vi "Voltage Based Speed Control (FPGA).vi"(0 "SpeedRead":fxp<+/-,20,5>, 5 "SpeedCtrl":fxp<+/-,20,5>, 7 "Speed?":bool, 9 "VoltCtrl":fxp<+/-,20,5>, 11 "SpeedCtrlRate":i16, 12 "SpeedStep":fxp<+/-,20,5>) -> (8 "VoltCtrlOut":fxp<+/-,21,6>)   [LabVIEW 2013]
uses:
  <vilib>/rvi/FXPMathLib/FxpDiv/subVIs/nifxpmath_Div_SimConfig.ctl
  <vilib>/rvi/Emulation/niFpgaSctlEmulationGetInTimedLoop.vi
  <vilib>/rvi/Emulation/niFpgaEmulationReportErrorSimple.vi
  <vilib>/rvi/Emulation/niFpgaGetClockAttributes.vi
  <vilib>/rvi/FXPMathLib/FxpDiv/simVIs/DllFxpDivTemp_sub.vi
  <vilib>/rvi/Emulation/niFpgaCriticalErrorInLSC.vi
  <vilib>/rvi/FXPMathLib/FxpSub/XNode/nifxpmath_Sub.xnode
  <vilib>/rvi/FXPMathLib/FxpDiv/XNode/nifxpmath_Div.xnode
  <vilib>/rvi/FXPMathLib/FxpMul/XNode/nifxpmath_Multiplier.xnode
  <vilib>/rvi/FXPMathLib/FxpAdd/XNode/nifxpmath_Add.xnode
  <vilib>/rvi/FXPMathLib/sim/FxpSim.dll
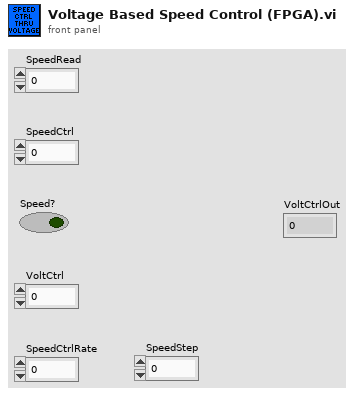
[diagram p1: front panel]
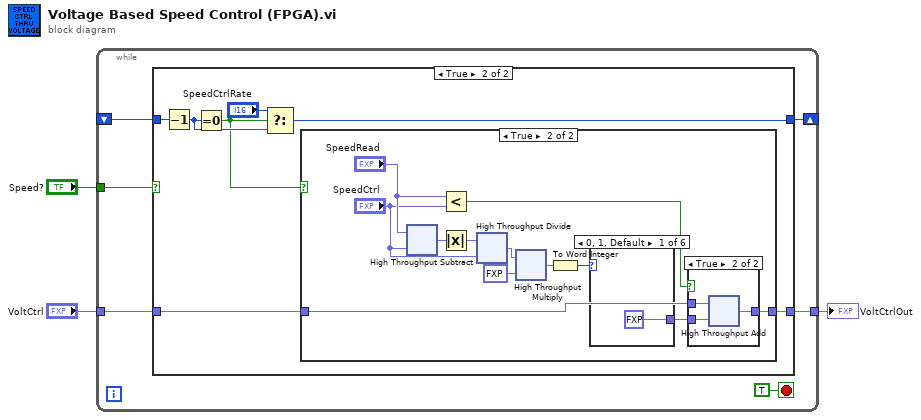
[diagram p0: block diagram]
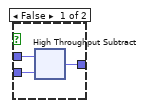
[diagram p4: hidden frame]
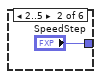
[diagram p5: hidden frame]
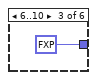
[diagram p6: hidden frame]
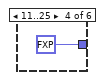
[diagram p7: hidden frame]
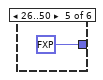
[diagram p8: hidden frame]
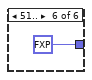
[diagram p9: hidden frame]
diagram:
  n1 = while {
    tunnel: "Speed?" -> [w9]
    tunnel: "VoltCtrl" -> [w8]
    tunnel: [w7] -> w1
    shift-right: [w4] -> _
    shift-left: _ -> [w5]
    stop <- TRUE stop-if-true
    n2 = case shown="True" w9 {
      tunnel: [w11 w12] -> w7
      tunnel: w8 -> [w11 w14]
      tunnel: w5 -> [_ w18]
      tunnel: [i16 0 ("SpeedCtrlRate") w15] -> w4
      frame False {
      }
      frame True {
        n3 = Decrement(x=w18) -> (x-1=w16:i16)
        n4 = Equal To 0?(x=w16) -> (x = 0?=w13:bool)
        n5 = Select(t="SpeedCtrlRate", s=w13, f=w16) -> (s? t:f=w15:i16)
        n6 = case shown="True" w13 {
          tunnel: w14 -> [w19 w21]
          tunnel: [w19 w22] -> w12
          frame False {
          }
          frame True {
            n7 = xnode "High Throughput Subtract"("x"="SpeedRead", "y"="SpeedCtrl") -> ("x-y"=w30:fxp<+/-,21,6>)
            n8 = Less?(x="SpeedRead", y="SpeedCtrl") -> (x < y?=w23:bool)
            n9 = Absolute Value(x=w30) -> (abs(x)=w29:fxp<+,21,6>)
            n10 = xnode "High Throughput Divide"("x"=w29, "y"="SpeedCtrl") -> ("x/y"=w27:fxp<+/-,22,22>)
            n11 = xnode "High Throughput Multiply"("x"=w27, "y"=fxp<+,7,7> 100.0) -> ("x*y"=w25:fxp<+/-,29,29>)
            n12 = To Word Integer(number=w25) -> (16bit integer=w24:i16)
            n13 = case shown="0, 1, Default" w24 {
              tunnel: [fxp<+/-,20,5> 0.0 ("y") "SpeedStep" fxp<+/-,20,5> 0.5 ("y") fxp<+/-,20,5> 2.0 ("y") fxp<+/-,20,5> 5.0 ("y") fxp<+/-,20,5> 10.0 ("y")] -> w20
              frame 0, 1, Default {
              }
              frame 2..5 {
              }
              frame 6..10 {
              }
              frame 11..25 {
              }
              frame 26..50 {
              }
              frame 51.. {
              }
            }
            n14 = case shown="True" w23 {
              tunnel: [w34 w37] -> w22
              tunnel: w21 -> [w33 w36]
              tunnel: w20 -> [w32 w35]
              frame False {
                n15 = xnode "High Throughput Subtract"("x"=w33, "y"=w32) -> ("x-y"=w34:fxp<+/-,21,6>)
              }
              frame True {
                n16 = xnode "High Throughput Add"("x"=w36, "y"=w35) -> ("x+y"=w37:fxp<+/-,21,6>)
              }
            }
          }
        }
      }
    }
  }
  "VoltCtrlOut" <- w1
